vi "Create.vi"   [LabVIEW 2020, in "Stream.lvlib" / "URLPattern.lvclass"]
uses:
  URLPattern.lvclass
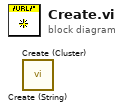
[diagram p0: block diagram]
diagram:
  n1 = call "Create (String).vi"() -> ()  [unwired: 10 in, 2 out]
  n2 = call "Create (Cluster).vi"() -> ()  [unwired: 10 in, 2 out]
